vi "ControlCenter.vi"() -> ()   [LabVIEW 2017]
uses:
  <vilib>/myRIO/Common/Instrument Driver Framework/myRIO v1.0/UART/vis/myRIO v1.0 Close UART.vi
  GlobalVarStop.vi
  <vilib>/myRIO/Common/Instrument Driver Framework/Utilities/vis/FPGA Ref Manager.vi
  <vilib>/myRIO/Common/Instrument Driver Framework/myRIO v1.0/myRIO v1.0 Reset FPGA.vi
  <vilib>/myRIO/Common/Instrument Driver Framework/myRIO v1.0/IRQ/vis/myRIO v1.0 IRQ Info FGV.vi
  <vilib>/myRIO/Common/Instrument Driver Framework/myRIO v1.0/IRQ/vis/myRIO v1.0 Timer IRQ Info FGV.vi
  <vilib>/myRIO/Common/Instrument Driver Framework/myRIO v1.0/IRQ/vis/myRIO v1.0 ISR Agent.vi
  <vilib>/myRIO/Instrument Drivers/Utilities/Utilities.lvlib
panel:
  out "Latitude":dbl(graph)
  out "Longitude":dbl(graph)
  out "Acquired\nFrames/s 2":dbl format="%.1g"
  out "Particle (x,y,pixels) 2":dbl[][](array[numeric]) format="%_2f"
  out "iteration 2":i32
  out "Sat":i32(graph)
  out "Satelites":string
  out "error out":errorcluster
  out "ReadMe":string
  out "Battery Level":dbl(slide) scale=8.5..12.0 scale format="%#_4g"
  out "hostKey1":i16
  out "iteration":i32
  out "iteration":i32
  out "iteration":i32
  out "iteration":i32
  out "Longitude (W)":string
  out "Latitude (N)":string
  out "Right":dbl format="%#_4g"
  out "Right":dbl
  out "Left":dbl format="%#_4g"
  out "Left":dbl
  out "Speed-R":i8(slide) min=-100 max=100 step=1 scale=-100.0..100.0
  out "Speed-L":i8(slide) min=-100 max=100 step=1 scale=-100.0..100.0
  in  "stop":bool
  in  "Decoration":bool
  in  "Decoration 2":bool
  in  "Decoration 3":bool
  in  "Decoration 4":bool
  in  "Decoration 5":bool
  in  "Decoration 6":bool
  # "ASEP Robot Control"
  # "Stop"
  # "Vision Control"
  # "Motor Driver Data"
  # "GPS Data"
  # "Motor Control"
  # "Keyboard Data"
  # "Temp (C)"
  # "Voltage (v)"
  # "Battery Level (v)"
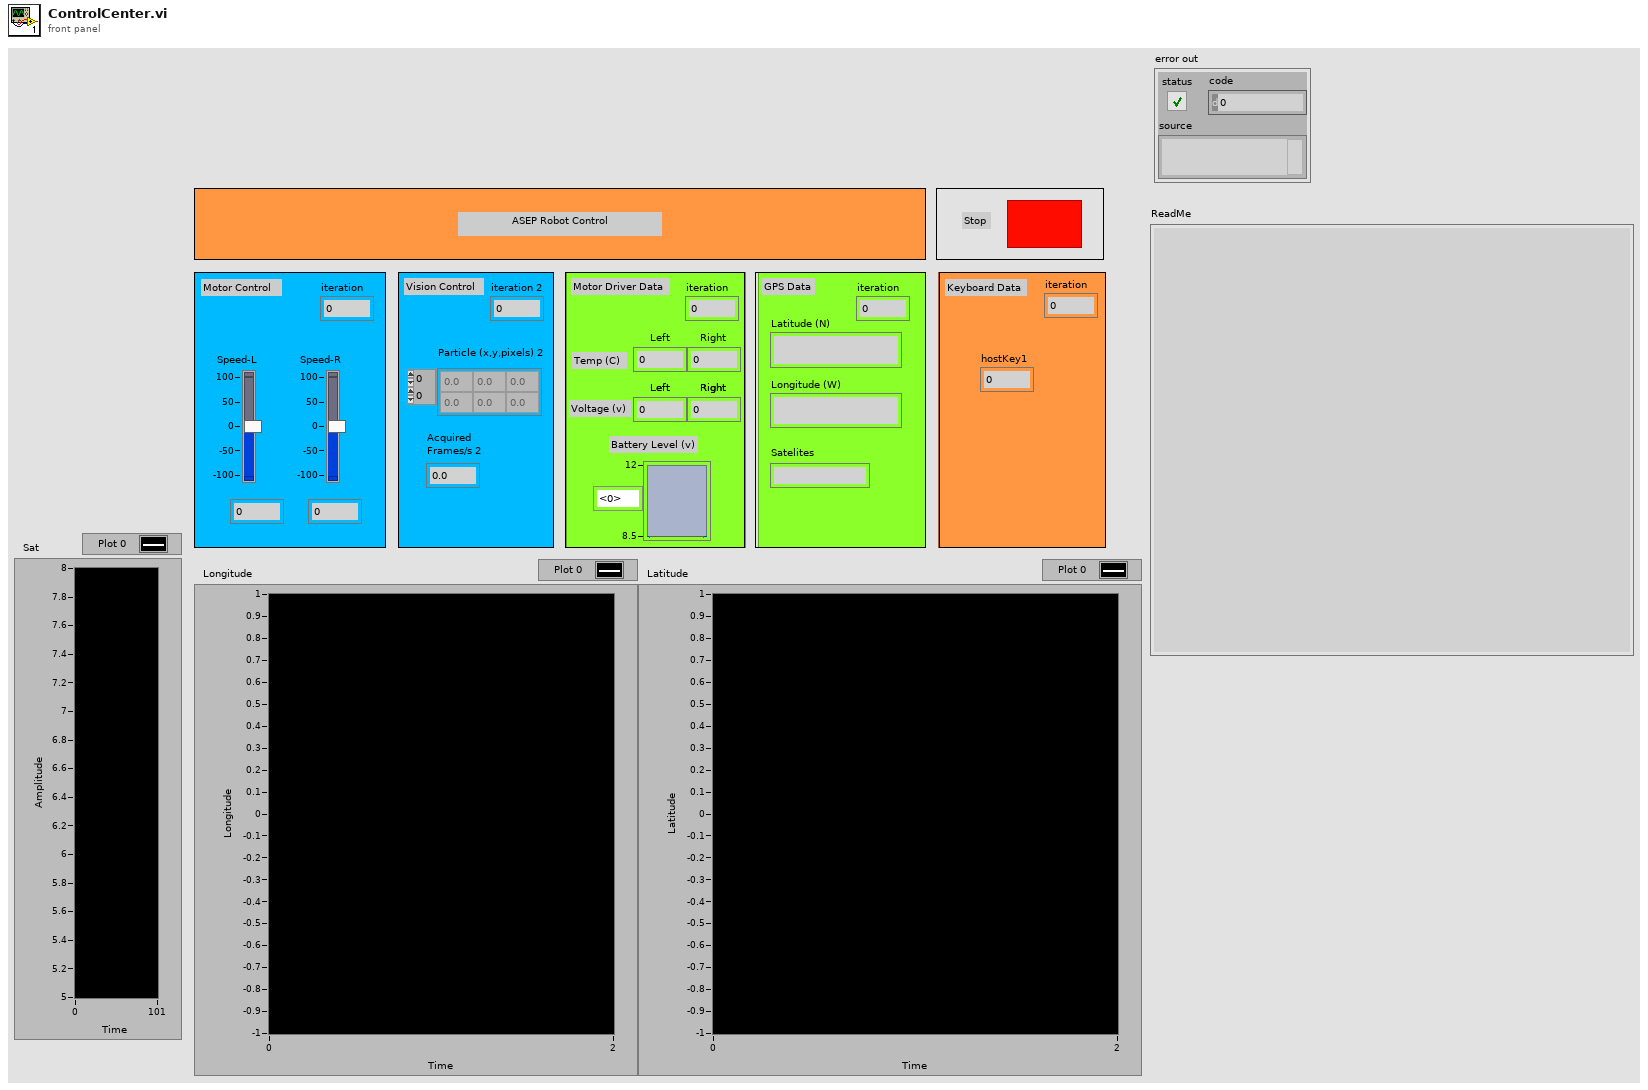
[diagram p1: front panel]
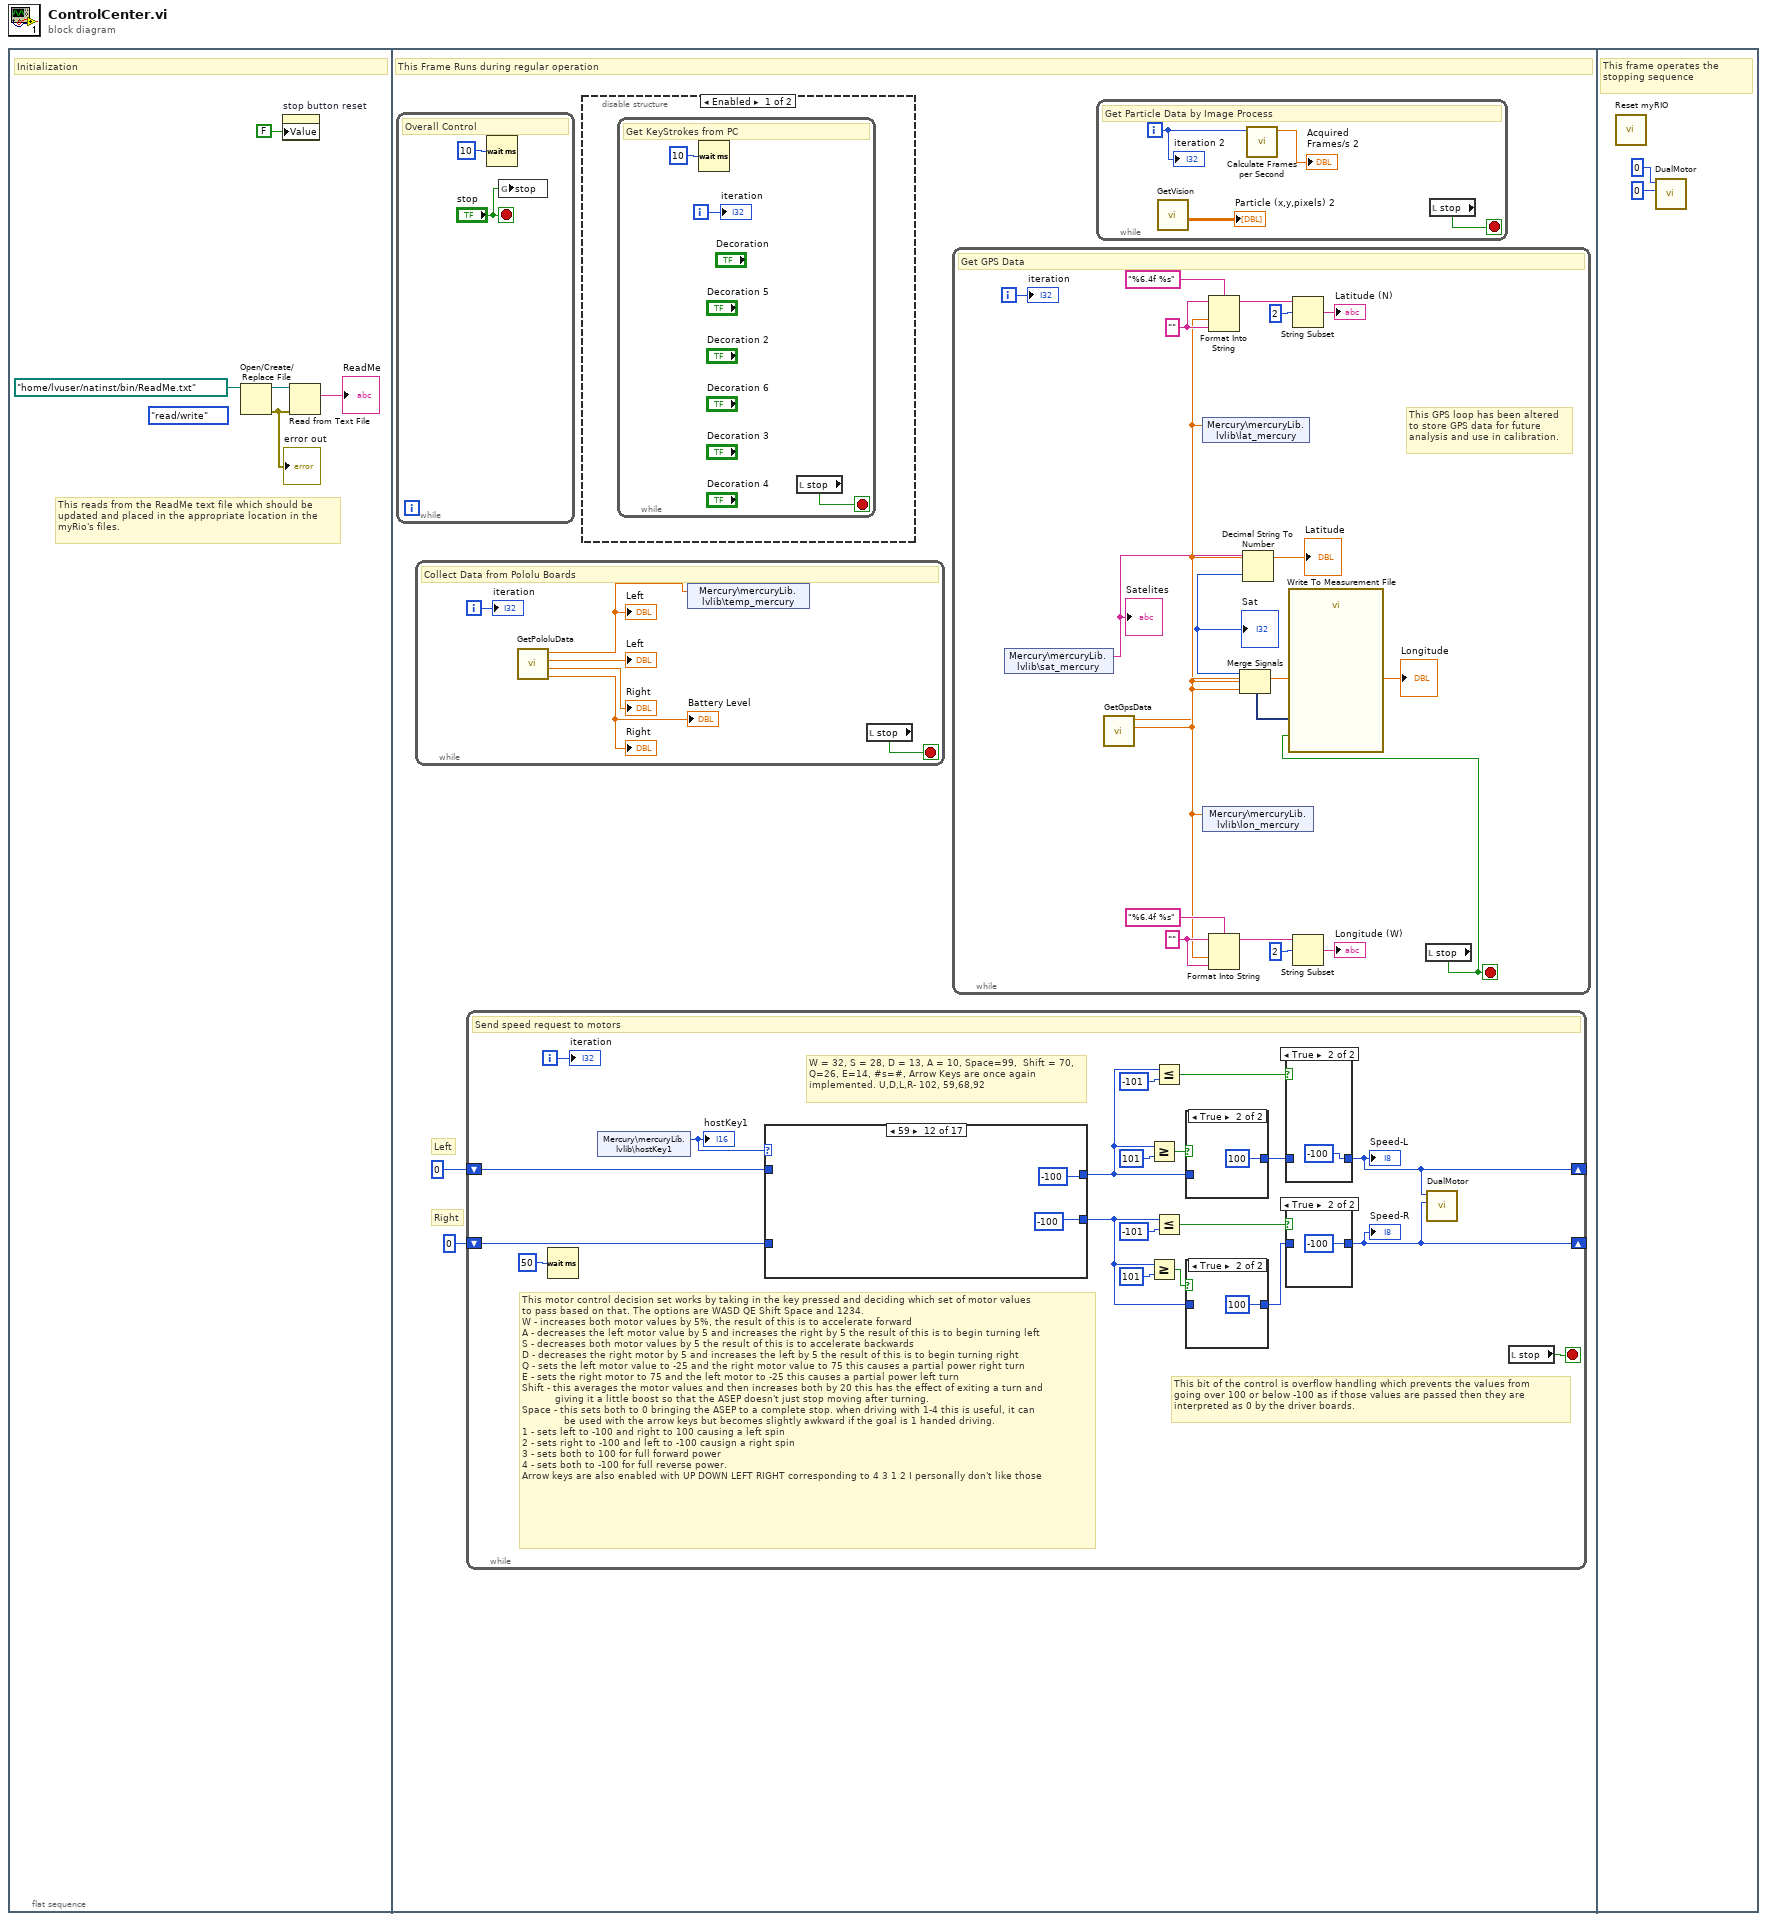
[diagram p0: block diagram]
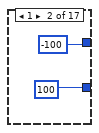
[diagram p8: hidden frame]
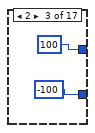
[diagram p9: hidden frame]
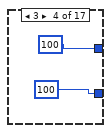
[diagram p10: hidden frame]
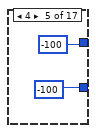
[diagram p11: hidden frame]
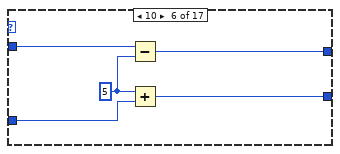
[diagram p12: hidden frame]
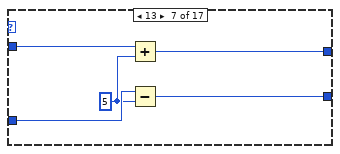
[diagram p13: hidden frame]
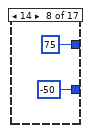
[diagram p14: hidden frame]
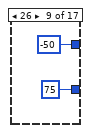
[diagram p15: hidden frame]
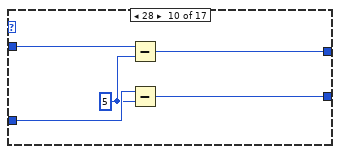
[diagram p16: hidden frame]
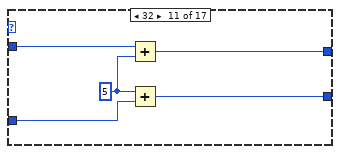
[diagram p17: hidden frame]
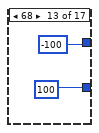
[diagram p18: hidden frame]
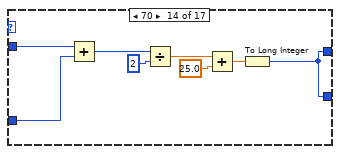
[diagram p19: hidden frame]
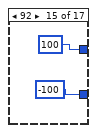
[diagram p20: hidden frame]
diagram:
  n1 = flat-sequence {
    frame #0 {
      (unwired) enum16{"read/write", "read-only", "write-only"}."read/write" ("access (0:read/write)")
      # "This reads from the ReadMe text file which should be\nupdated and placed in the appropriate location in the\nmyRio's files."
      # "Initialization"
      n2 = Open/Create/Replace File(file path (use dialog)=path "/home/lvuser/natinst/bin/ReadMe.txt" ("file (use dialog)")) -> (refnum out=w3:refnum<file>, error out=w4:errorcluster)  [unwired: 5 in, 1 out]
      "error out" <- w4
      n3 = property on="stop button reset" class="Bool (strict)"("Value"=FALSE ("stop")) -> ()  [unwired: 2 in, 2 out]
      n4 = Read from Text File(file (use dialog)=w3, error in=w4) -> (text=→"ReadMe":string)  [unwired: 2 in, 3 out]
    }
    frame #1 {
      # "Right"
      # "Left"
      # "This Frame Runs during regular operation"
      n5 = while {
        stop <- "stop" stop-if-true
        # "Overall Control"
        n6 = Wait (ms)(milliseconds to wait=u32 10) -> ()  [unwired: 1 out]
        n7 = global write "GlobalVarStop.vi" "stop"("stop") -> ()
      }
      n8 = while {
        i -> [w35]
        stop <- w37 stop-if-true
        # "Collect Data from Pololu Boards"
        n9 = call "GetPololuData.vi"() -> ("Right Board Voltage"=→"Right" →"Battery Level":dbl, "Right Board Temp"=→"Right":dbl, "Left Board Voltage"=→"Left":dbl, "Left Board Temp"=w36:dbl)  [unwired: 8 in]
        "Left" <- w36
        n10 = shared-variable "Mercury\\mercuryLib.lvlib\\temp_mercury"(w36) -> ()  [unwired: 1 in, 1 out]
        n11 = local read "stop"() -> (w37:bool)
        "iteration" <- w35
      }
      n12 = while {
        shift-right: [w41] -> _
        shift-left: 0 -> [w56]
        shift-right: [w40] -> _
        shift-left: 0 -> [w55]
        i -> [w58]
        stop <- w59 stop-if-true
        # "This bit of the control is overflow handling which prevents the values from \ngoing over 100 or below -100 as if those values are passed then they are \ninterpreted as 0 by the driver boards."
        # "This motor control decision set works by taking in the key pressed and deciding which set of motor values\nto pass based on that. The options are WASD QE Shift Space and 1234. \nW - increases both motor values by 5%, the result of this is to accelerate forward\nA - decreases the left motor value by 5 and increases the right by 5 the result of this is to begin turning left\nS - decreases both motor values by 5 the result of this is to accelerate backwards\nD - decreases the right motor by 5 and increases the left by 5 the result of this is to begin turning right\nQ - sets the left motor value to -25 and the right motor value to 75 this causes a partial power right turn\nE - sets the right motor to 75 and the left motor to -25 this causes a partial power left turn\nShift - this averages the motor values and then increases both by 20 this has the effect of exiting a turn and\n           giving it a little boost so that the ASEP doesn't just stop moving after turning. \nSpace - this sets both to 0 bringing the ASEP to a complete stop. when driving with 1-4 this is useful, it can \n              be used with the arrow keys but becomes slightly awkward if the goal is 1 handed driving. \n1 - sets left to -100 and right to 100 causing a left spin\n2 - sets right to -100 and left to -100 causign a right spin\n3 - sets both to 100 for full forward power\n4 - sets both to -100 for full reverse power.\nArrow keys are also enabled with UP DOWN LEFT RIGHT corresponding to 4 3 1 2 I personally don't like those"
        # "W = 32, S = 28, D = 13, A = 10, Space=99,  Shift = 70, Q=26, E=14, #s=#, Arrow Keys are once again implemented. U,D,L,R- 102, 59,68,92"
        # "Send speed request to motors"
        n13 = Wait (ms)(milliseconds to wait=u32 50) -> ()  [unwired: 1 out]
        n14 = shared-variable "Mercury\\mercuryLib.lvlib\\hostKey1"() -> (w57:i16)  [unwired: 1 in, 1 out]
        "hostKey1" <- w57
        n15 = case shown="59" w57 {
          tunnel: [w68 100 -100 100 -100 w81 w83 -50 75 w93 w98 -100 100 w109 -100 w116 100] -> w43
          tunnel: [w69 -100 100 100 -100 w78 w86 75 -50 w95 w97 -100 -100 w109 100 w116 100] -> w50
          tunnel: w56 -> [w69 _ _ _ _ w79 w87 _ _ w96 w101 _ _ w113 _ _ _]
          tunnel: w55 -> [w68 _ _ _ _ w82 w85 _ _ w94 w99 _ _ w112 _ _ _]
          frame 0, Default {
          }
          frame 1 {
          }
          frame 2 {
          }
          frame 3 {
          }
          frame 4 {
          }
          frame 10 {
            w80 = 5
            n16 = Subtract(x=w79, y=w80) -> (x-y=w78:i32)
            n17 = Add(x=w80, y=w82) -> (x+y=w81:i32)
          }
          frame 13 {
            w84 = 5
            n18 = Add(x=w87, y=w84) -> (x+y=w86:i32)
            n19 = Subtract(x=w85, y=w84) -> (x-y=w83:i32)
          }
          frame 14 {
          }
          frame 26 {
          }
          frame 28 {
            w92 = 5
            n20 = Subtract(x=w96, y=w92) -> (x-y=w95:i32)
            n21 = Subtract(x=w94, y=w92) -> (x-y=w93:i32)
          }
          frame 32 {
            w100 = 5
            n22 = Add(x=w101, y=w100) -> (x+y=w97:i32)
            n23 = Add(x=w100, y=w99) -> (x+y=w98:i32)
          }
          frame 59 {
          }
          frame 68 {
          }
          frame 70 {
            n24 = Add(x=w113, y=w112) -> (x+y=w111:i32)
            n25 = Divide(x=w111, y=2) -> (x/y=w108:dbl)
            n26 = Add(x=w108, y=25.0) -> (x+y=w107:dbl)
            n27 = To Long Integer(number=w107) -> (32bit integer=w109:i32)
          }
          frame 92 {
          }
          frame 99 {
            w116 = 0
          }
          frame 102 {
          }
        }
        n28 = Greater Or Equal?(x=w50, y=101) -> (x >= y?=w51:bool)
        n29 = Greater Or Equal?(x=w43, y=101) -> (x >= y?=w44:bool)
        n30 = Less Or Equal?(x=w50, y=-101) -> (x <= y?=w48:bool)
        n31 = Less Or Equal?(x=w43, y=-101) -> (x <= y?=w45:bool)
        n32 = case shown="True" w51 {
          tunnel: [w66 100 ("y")] -> w49
          tunnel: w50 -> [w66 _]
          frame False {
          }
          frame True {
          }
        }
        n33 = case shown="True" w44 {
          tunnel: [w60 100 ("y")] -> w42
          tunnel: w43 -> [w60 _]
          frame False {
          }
          frame True {
          }
        }
        n34 = case shown="True" w48 {
          tunnel: [w64 -100 ("y")] -> w41
          tunnel: w49 -> [w64 _]
          frame False {
          }
          frame True {
          }
        }
        "Speed-L" <- w41
        n35 = case shown="True" w45 {
          tunnel: [w62 -100 ("y")] -> w40
          tunnel: w42 -> [w62 _]
          frame False {
          }
          frame True {
          }
        }
        "Speed-R" <- w40
        n36 = call "DualMotor.vi"("Speed-R"=w40, "Speed-L"=w41) -> ()  [unwired: 10 in]
        n37 = local read "stop"() -> (w59:bool)
        "iteration" <- w58
      }
      n38 = disable-structure shown="Enabled" {
        frame Enabled {
          n39 = while {
            i -> [w13]
            stop <- w14 stop-if-true
            # "Get KeyStrokes from PC"
            n40 = Wait (ms)(milliseconds to wait=u32 10) -> ()  [unwired: 1 out]
            n41 = local read "stop"() -> (w14:bool)
            "iteration" <- w13
          }
        }
        frame Disabled {
        }
      }
      n42 = while {
        i -> [w31]
        stop <- w15 stop-if-true
        w27 = "" ("initial string")
        w28 = "" ("initial string")
        # "This GPS loop has been altered\nto store GPS data for future\nanalysis and use in calibration."
        # "Get GPS Data"
        n43 = shared-variable "Mercury\\mercuryLib.lvlib\\sat_mercury"() -> (w22:string)  [unwired: 1 in, 1 out]
        "Satelites" <- w22
        n44 = call "GetGpsData.vi"() -> ("Latitude (N)"=w17:dbl, "Longitude (W)"=w18:dbl)  [unwired: 8 in]
        "Latitude" <- w17
        "Longitude" <- w18
        n45 = shared-variable "Mercury\\mercuryLib.lvlib\\lat_mercury"(w17) -> ()  [unwired: 1 in, 1 out]
        n46 = shared-variable "Mercury\\mercuryLib.lvlib\\lon_mercury"(w18) -> ()  [unwired: 1 in, 1 out]
        n47 = Format Into String(format string="%6.4f %s", initial string=w27, w17, w27) -> (resulting string=w26:string)  [unwired: 1 in, 1 out]
        n48 = Format Into String(format string="%6.4f %s", initial string=w28, w18, w28) -> (resulting string=w23:string)  [unwired: 1 in, 1 out]
        n49 = Decimal String To Number(string=w22) -> (number=w16:i32)  [unwired: 2 in, 1 out]
        "Sat" <- w16
        n50 = Merge Signals(w16, w17, w18) -> (w19:dynamicdata)
        n51 = String Subset(string=w26, offset (0)=2) -> (substring=→"Latitude (N)":string)  [unwired: 1 in]
        n52 = String Subset(string=w23, offset (0)=2) -> (substring=→"Longitude (W)":string)  [unwired: 1 in]
        n53 = local read "stop"() -> (w15:bool)
        n54 = call "Write To Measurement File"("Signals"=w19, "Flush? (T)"=w15) -> ()  [unwired: 15 in, 3 out]
        "iteration" <- w31
      }
      n55 = while {
        i -> [w10]
        stop <- w8 stop-if-true
        # "Get Particle Data by Image Process"
        n56 = call "GetVision.vi"() -> ("Particle Measurements\n         X             Y           area"=→"Particle (x,y,pixels) 2":dbl[][])  [unwired: 11 in]
        n57 = call <vilib>:"Calculate Frames per Second.vi"("Buffer Number"=w10) -> ("Acquired Frames/s"=→"Acquired\nFrames/s 2":dbl)  [unwired: 8 in, 2 out]
        n58 = local read "stop"() -> (w8:bool)
        "iteration 2" <- w10
      }
    }
    frame #2 {
      # "This frame operates the stopping sequence"
      n59 = call <vilib>:"Reset myRIO.vi"() -> ()  [unwired: 11 in, 1 out]
      n60 = call "DualMotor.vi"("Speed-R"=i8 0 ("Speed-R 2"), "Speed-L"=i8 0 ("Speed-L 2")) -> ()  [unwired: 10 in]
    }
  }
